vi "Global vars.vi"() -> ()   [LabVIEW 2018]
panel:
  out "Phase 4":dbl
  out "Phase 3":dbl
  out "Phase 2":dbl
  out "Phase 1":dbl
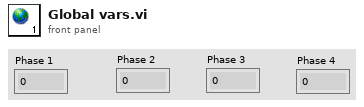
[diagram p1: front panel]
diagram:
